vi "write hitchart data.vi"(5 "channel":i32=-1, 7 "Histogram cluster":T1 {"ID" format="ch %d"}, 8 "error in (no error)":errorcluster, 11 "Hit charts":T2) -> (0 "error out":errorcluster, 3 "Hit charts":T2)   [LabVIEW 2016]
uses:
  Typedefs/Hit chart cluster refnum.ctl
  Typedefs/HitChart.ctl
panel:
  # "Leave Channel unwired to use the channel index\nin the supplied chart"
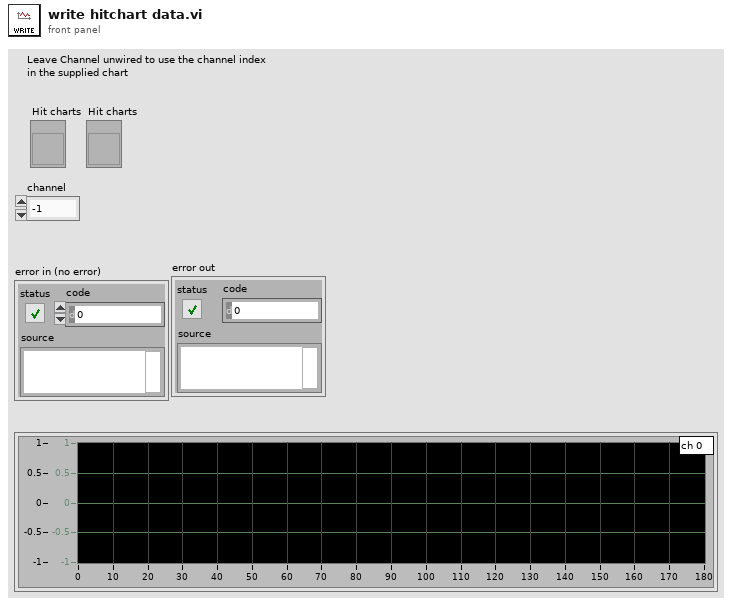
[diagram p1: front panel]
types:
  T1 = typedef "HitChart.ctl" = cluster{"Waveform Chart":cluster{"Coincidences":dbl, "Non-coincidences":dbl, "Ratio":dbl, "Total hits":dbl}[], "Last update timestamp":timestamp, "Resolution(s)":dbl, "nondisplayed coincs":i32, "nondisplayed noncoincs":i32, "Last upd":i64, "ID":i8}
  T2 = typedef "Hit chart cluster refnum.ctl" = refnum<vi>
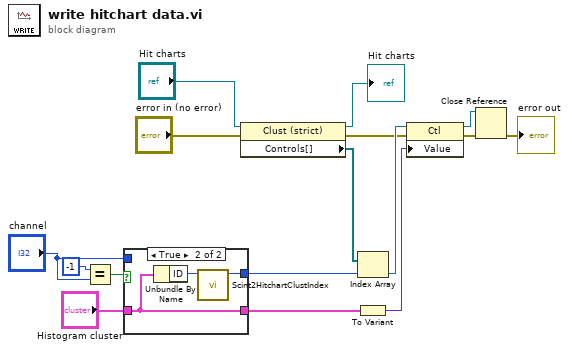
[diagram p0: block diagram]
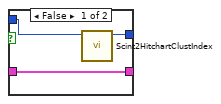
[diagram p2: hidden frame]
diagram:
  n1 = Equal?(x=-1, y="channel") -> (x = y?=w1:bool)
  n2 = case shown="True" w1 {
    tunnel: "channel" -> [w19 _]
    tunnel: [w18 w21] -> w8
    tunnel: [w17 w22] -> w5
    tunnel: "Histogram cluster" -> [w17 w22]
    frame False {
      n3 = call "Scint2HitchartClustIndex.vi"("Channel"=w19) -> ("Numeric"=w18:i8)  [unwired: 10 in]
    }
    frame True {
      n4 = Unbundle By Name(w22) -> ("ID"=w20:i8)
      n5 = call "Scint2HitchartClustIndex.vi"("Channel"=w20) -> ("Numeric"=w21:i8)  [unwired: 10 in]
    }
  }
  n6 = property class="Clust (strict)"(reference="Hit charts", error in="error in (no error)") -> (reference out=→"Hit charts":T2, error out=w9:errorcluster, "Controls[]"=w16:refnum<vi>[])
  n7 = Index Array(array=w16, index=w8) -> (element=w10:refnum<vi>)
  n8 = To Variant(anything=w5) -> (Variant=w12:variant)
  n9 = property class="Ctl"(reference=w10, error in=w9, "Value"=w12) -> (reference out=w13:refnum<vi>, error out=w14:errorcluster)
  n10 = Close Reference(reference=w13, error in (no error)=w14) -> (error out=→"error out":errorcluster)
